vi "BooleanRise.vi"(11 "Test Mode On":bool) -> (3 "Boolean":bool)   [LabVIEW 2017]
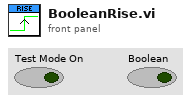
[diagram p1: front panel]
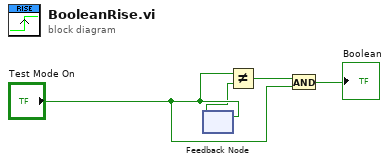
[diagram p0: block diagram]
diagram:
  n1 = feedback #1() -> (w1:bool)  [unwired: 1 in]
  n2 = feedback-in #1("Test Mode On") -> ()
  n3 = Not Equal?(x="Test Mode On", y=w1) -> (x != y?=w2:bool)
  n4 = And(x=w2, y="Test Mode On") -> (x .and. y?=→"Boolean":bool)
